vi "Set TEC Enable.vi"(8 "error in":errorcluster, 11 "cPAS in":refnum<class "cPAS.lvclass">) -> (0 "error out":errorcluster, 3 "cPAS out":refnum<class "cPAS.lvclass">)   [LabVIEW 2015, in "cPAS.lvclass"]
uses:
  cPAS.lvclass
  cPAS.lvclass/cPAS.ctl
  <vilib>/DAQmx/write.llb/DAQmx Write (Digital 1D Bool NChan 1Samp 1Line).vi
  <vilib>/DAQmx/miscellaneous.llb/DAQmx Fill In Error Info.vi
  Reusable/Instrument/Instrument.lvclass
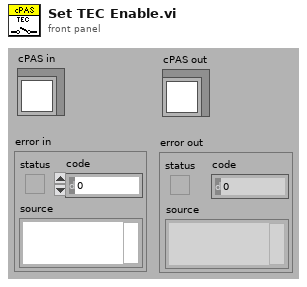
[diagram p1: front panel]
types:
  T1 = cluster{"Cell 1":bool, "Cell 2":bool, "Cell 3":bool, "Cell 4":bool, "Cell 5":bool}
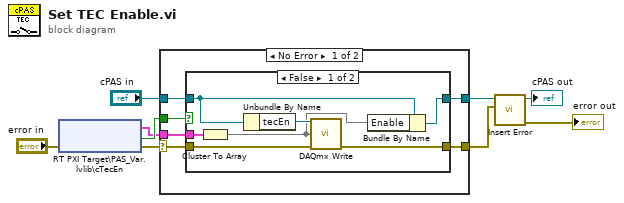
[diagram p0: block diagram]
diagram:
  n1 = shared-variable "RT PXI Target\\PAS_Var.lvlib\\cTecEn"(error in="error in") -> (w8:T1, error out=w5:errorcluster, w9:bool)  [unwired: 1 in]
  n2 = case shown="No Error" w5 {
    selector: w5 -> [w10 w26]
    tunnel: w9 -> [w15 _]
    tunnel: w8 -> [w14 _]
    tunnel: "cPAS in" -> [w13 w25]
    tunnel: [w12 w25] -> w4
    tunnel: [w11 w26] -> w2
    frame No Error {
      n3 = case shown="False" w15 {
        tunnel: w13 -> [w18 w24]
        tunnel: [w16 w24] -> w12
        tunnel: [w19 w23] -> w11
        tunnel: w10 -> [w20 w23]
        tunnel: w14 -> [w21 _]
        frame False {
          n4 = Cluster To Array(cluster=w21) -> (array=w17:bool[])
          n5 = Unbundle By Name(w18) -> ("tecEn"=w22:refnum<k21>)
          n6 = call-poly <vilib>:"DAQmx Write.vi"("task/channels in"=w22, "data"=w17, "error in"=w20) -> ("error out"=w19:errorcluster)  [unwired: 10 in, 2 out]
          n7 = Bundle By Name(cluster=w18, "Enable"=w17) -> (w16:refnum<class "cPAS.lvclass">)
        }
        frame True {
        }
      }
    }
    frame Error {
    }
  }
  n8 = call "Insert Error.vi"("err"=w2, "Instrument in"=w4) -> ("error out"=→"error out":errorcluster, "Instrument out"=→"cPAS out":refnum<class "cPAS.lvclass">)  [unwired: 7 in, 1 out]
